vi "Main - On Load.vi"(8 "error in (no error)":errorcluster, 11 "Device Item Ref in":T1 format="%.0x") -> (0 "error out":errorcluster, 3 "Device Item Ref out":T1 format="%.0x")   [LabVIEW 2017, in "Scan Engine Custom Device.lvlib"]
uses:
  Scan Engine Custom Device.lvlib
  <vilib>/NI Veristand/Custom Device API/Custom Device Item Ref.ctl
  <vilib>/NI Veristand/Custom Device API/Custom Device Channel.ctl
  <vilib>/NI Veristand/Custom Device API/Custom Device Channel Type.ctl
  NationalInstruments.VeriStand.SystemDefinitionAPI
  Globals/Scan Engine GUIDs.vi
  Globals/Property Strings.vi
  <vilib>/NI Veristand/Custom Device Tools/Custom Device Utility Library/NI VeriStand - Search for All Items by GUID.vi
  <vilib>/NI Veristand/Custom Device API/Get Item Property (U32).vi
  Globals/String Constants.vi
  <vilib>/NI Veristand/Custom Device API/Set Item Property (Boolean).vi
  <vilib>/NI Veristand/Custom Device API/Custom Device API.lvlib
  <vilib>/NI Veristand/Custom Device Tools/Custom Device Utility Library/Custom Device Utility Library.lvlib
  Modules.lvlibp/RSI Module/RSI Module.lvclass
  Modules.lvlibp
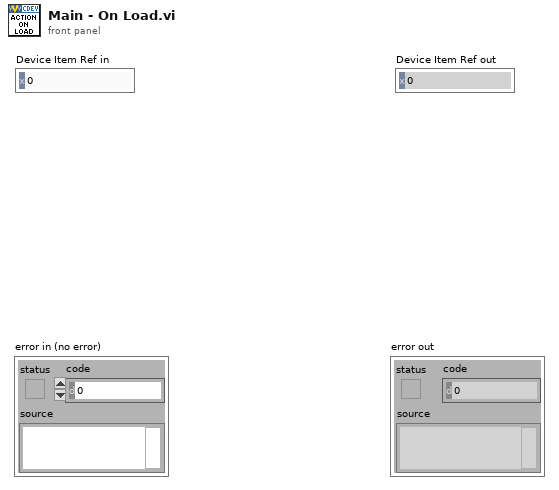
[diagram p1: front panel]
types:
  T1 = typedef "Custom Device API.lvlib/Custom Device Item Ref.ctl" = u64
  T2 = typedef "Custom Device API.lvlib/Custom Device Channel.ctl" = cluster{"Type":T3, "Units":string, "Default Value":dbl, "Faultable":bool, "Scalable":bool}
  T3 = typedef "Custom Device API.lvlib/Custom Device Channel Type.ctl" = enum16{"Input", "Output"}
  T4 = typedef "Modules.lvlibp/Custom Device API.lvlib/Custom Device Item Ref.ctl" = u64
  T5 = typedef "Modules.lvlibp/RSI Module.lvclass/Module Models.ctl" = enum16{"Empty", "NI 9201", "NI 9203", "NI 9205", "NI 9206", "NI 9207", "NI 9208", "NI 9211", "NI 9212", "NI 9213", "NI 9214", "NI 9215", "NI 9217", "NI 9219", "NI 9220", "NI 9221", "NI 9222", "NI 9223", "NI 9224", "NI 9225", "NI 9227", "NI 9229", "NI 9233", "NI 9234", "NI 9235", "NI 9236", "NI 9237", "NI 9239", "NI 9242", "NI 9244", "NI 9263", "NI 9264", "NI 9265", "NI 9266", "NI 9269", "NI 9375", "NI 9401", "NI 9402", "NI 9403", "NI 9411", "NI 9421", "NI 9422", "NI 9423", "NI 9425", "NI 9426", "NI 9435", "NI 9437", "NI 9472", "NI 9474", "NI 9475", "NI 9476", "NI 9477", "NI 9478", "NI 9481", "NI 9482", "NI 9485"}
  T6 = typedef "Modules.lvlibp/RSI Module.lvclass/Slot Settings.ctl" = cluster{"Slot":u32, "EtherCAT?":bool}
  T7 = typedef "Custom Device API.lvlib/Custom Device Item Info.ctl" = cluster{"Name":string, "Is Channel":bool, "GUID":string, "Is Waveform":bool}
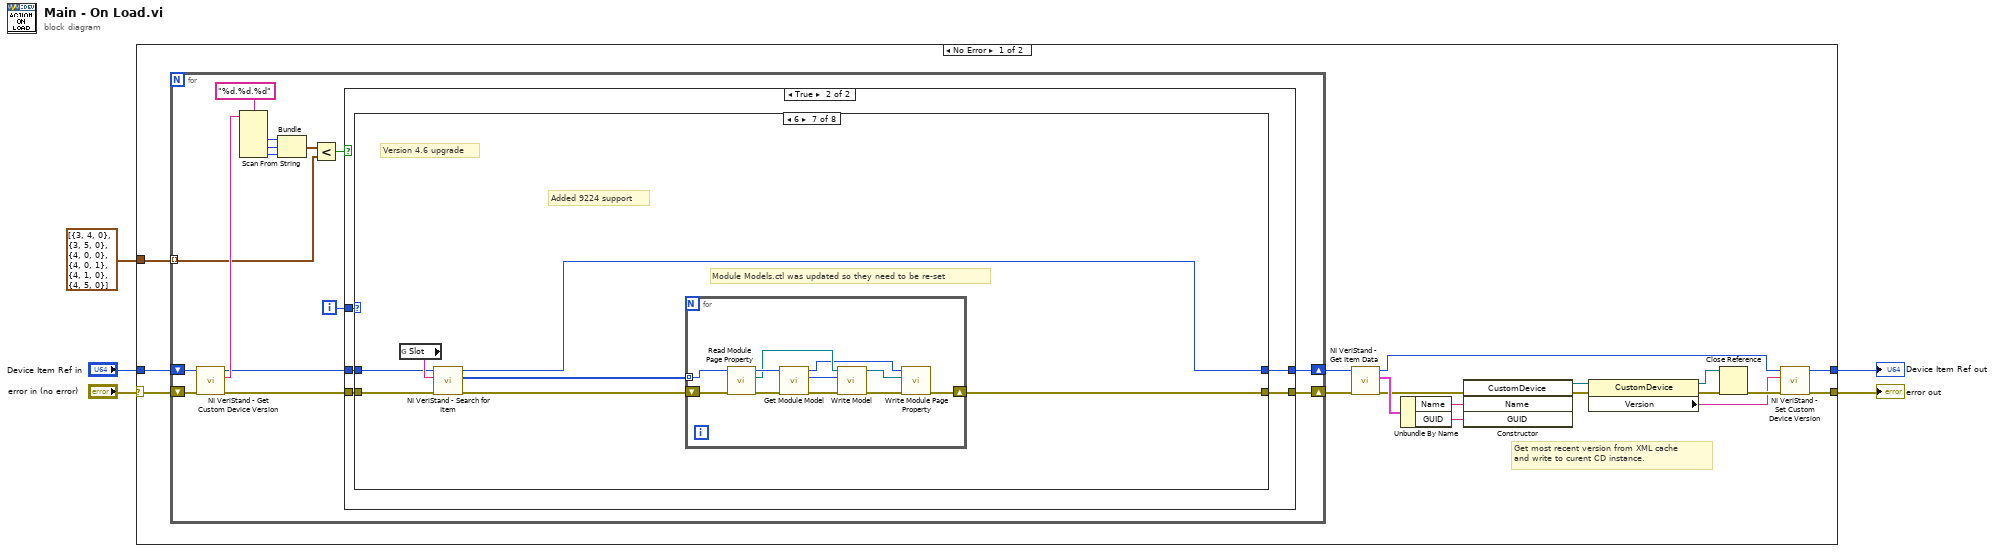
[diagram p0: block diagram]
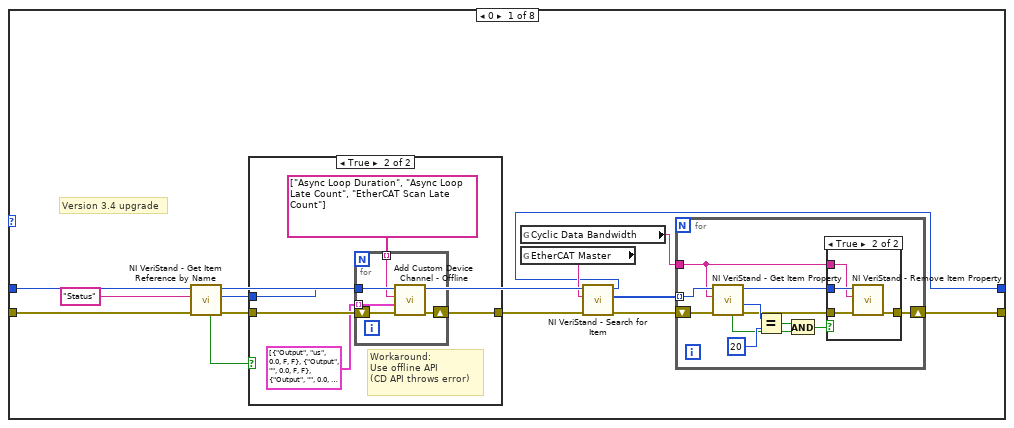
[diagram p3: hidden frame]
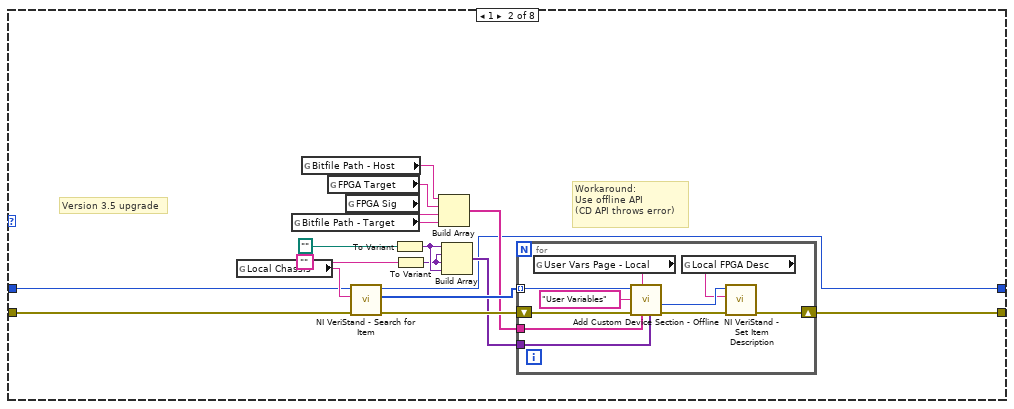
[diagram p6: hidden frame]
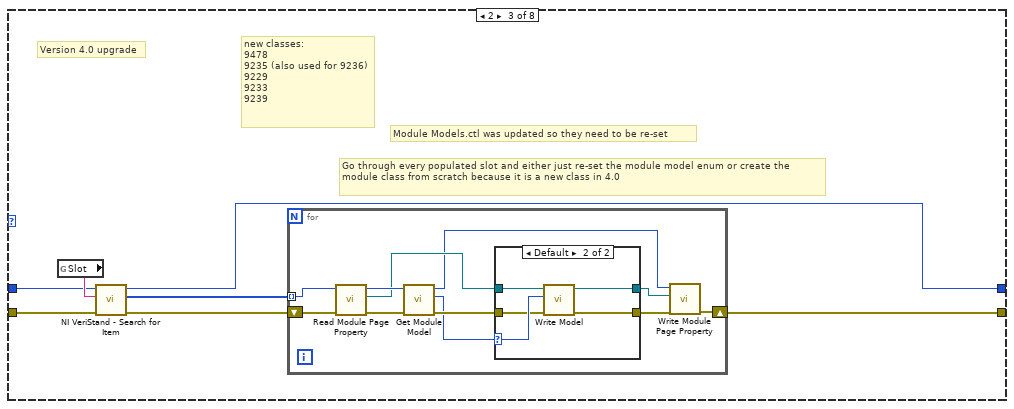
[diagram p7: hidden frame]
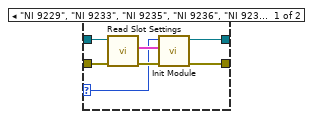
[diagram p8: hidden frame]
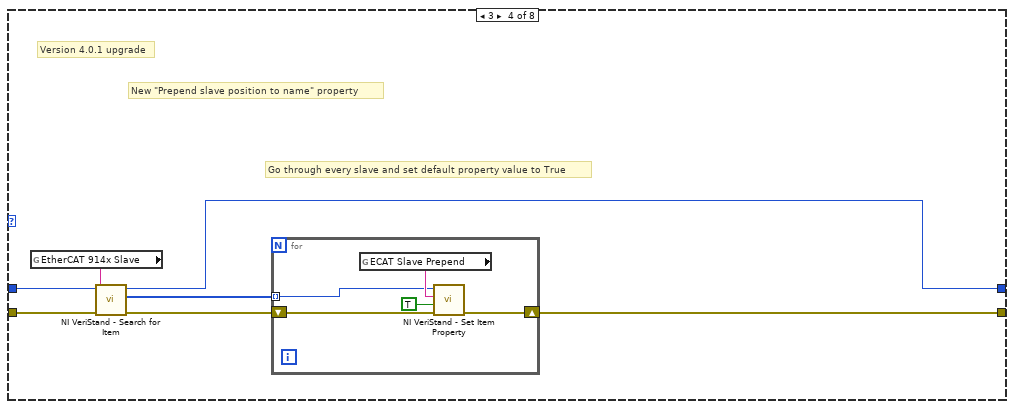
[diagram p9: hidden frame]
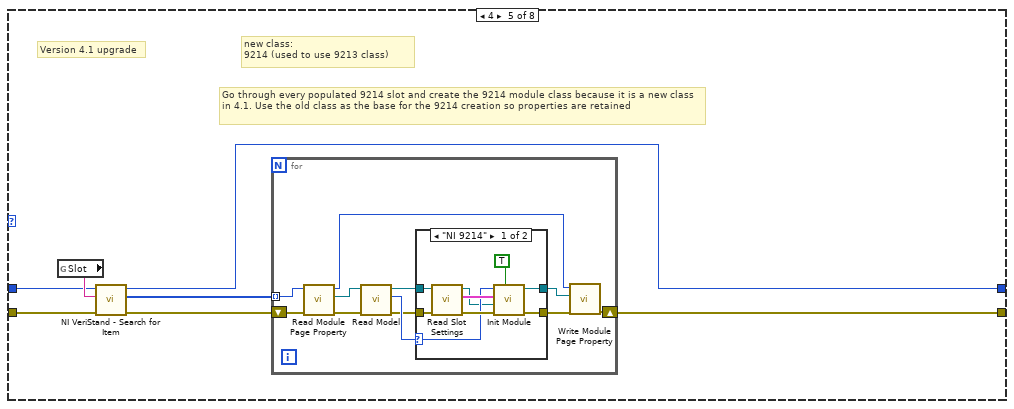
[diagram p10: hidden frame]
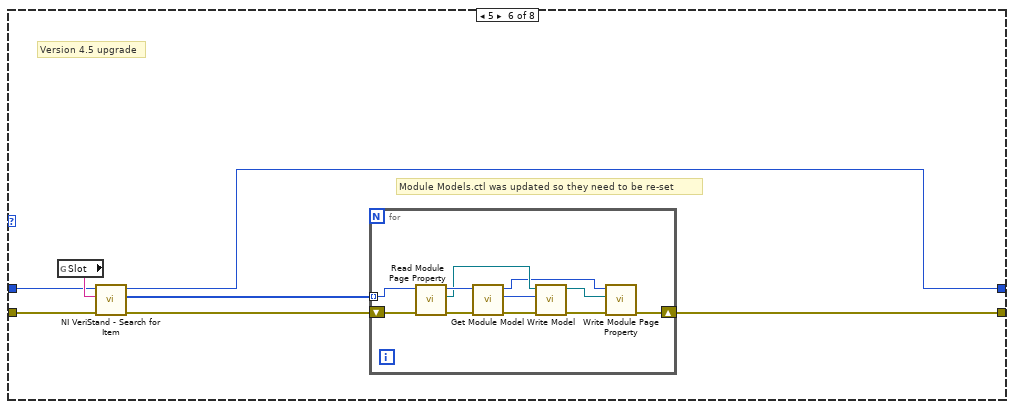
[diagram p12: hidden frame]
diagram:
  n1 = case shown="No Error" "error in (no error)" {
    selector: "error in (no error)" -> [w23 w224]
    tunnel: [w6 w224] -> w3
    tunnel: "Device Item Ref in" -> [w22 w223]
    tunnel: [w7 w223] -> w2
    tunnel: cluster{i32, i32, i32}[] [{3, 4, 0}, {3, 5, 0}, {4, 0, 0}, {4, 0, 1}, {4, 1, 0}, {4, 5, 0}] -> [w21 _]
    frame No Error {
      # "Get most recent version from XML cache\nand write to curent CD instance."
      n2 = for {
        shift-right: [w29] -> w19
        shift-left: w23 -> [w34]
        shift-right: [w27] -> w20
        shift-left: w22 -> [w33]
        tunnel: w21 -> [w24] mode=indexing
        i -> [w26]
        n3 = call <vilib>:"NI VeriStand - Get Custom Device Version.vi"("error in (no error)"=w34, "Device Ref in"=w33) -> ("error out"=w30:errorcluster, "Value"=w32:string, "Device Ref out"=w28:T1)  [unwired: 7 in]
        n4 = Scan From String(format string="%d.%d.%d", input string=w32) -> (output 1=w36:i32, output 2=w37:i32, output 3=w25:i32)  [unwired: 5 in, 3 out]
        n5 = Bundle(w36, w37, w25) -> (w38:cluster{i32, i32, i32})  [unwired: 1 in]
        n6 = Less?(x=w38, y=w24) -> (x < y?=w31:bool)
        n7 = case shown="True" w31 {
          tunnel: w30 -> [w40 w45]
          tunnel: [w40 w44] -> w29
          tunnel: w28 -> [w39 w41]
          tunnel: [w39 w42] -> w27
          tunnel: w26 -> [_ w43]
          frame False {
          }
          frame True {
            n8 = case shown="6" w43 {
              tunnel: w45 -> [w46 w89 w116 w146 w158 w187 w205 w222]
              tunnel: [w52 w88 w115 w145 w157 w186 w204 w222] -> w44
              tunnel: [w54 w87 w114 w144 w156 w185 w203 w221] -> w42
              tunnel: w41 -> [w47 w90 w117 w147 w159 w188 w206 w221]
              frame 0 {
                # "Version 3.4 upgrade"
                n9 = call <vilib>:"NI VeriStand - Get Item Reference by Name.vi"("error in (no error)"=w46, "Item Name"="Status" ("Section Name"), "Parent Ref in"=w47) -> ("error out"=w50:errorcluster, "Item Ref"=w49:T1, "Parent Ref out"=w58:T1, "Found"=w48:bool)  [unwired: 5 in]
                n10 = case shown="True" w48 {
                  tunnel: w49 -> [_ w65]
                  tunnel: w50 -> [w60 w64]
                  tunnel: [w60 w63] -> w59
                  frame False {
                  }
                  frame True {
                    # "Workaround:\nUse offline API\n(CD API throws error)"
                    n11 = for {
                      tunnel: w65 -> [w68]
                      shift-right: [w70] -> w63
                      shift-left: w64 -> [w69]
                      tunnel: T2[] [{"Type"=enum."Output", "Units"="us", "Default Value"=0.0, "Faultable"=FALSE, "Scalable"=FALSE}, {"Type"=enum."Output", "Units"="", "Default Value"=0.0, "Faultable"=FALSE, "Scalable"=FALSE}, {"Type"=enum."Output", "Units"="", "Default Value"=0.0, "Faultable"=FALSE, "Scalable"=FALSE}] -> [w66] mode=indexing
                      tunnel: string[] ["Async Loop Duration", "Async Loop Late Count", "EtherCAT Scan Late Count"] -> [w67] mode=indexing
                      n12 = call "Add Custom Device Channel - Offline.vi"("error in (no error)"=w69, "Channel"=w66, "Channel Name"=w67, "Parent Ref in"=w68) -> ("error out"=w70:errorcluster)  [unwired: 4 in, 3 out]
                    }
                  }
                }
                n13 = global read "Property Strings.vi" "Cyclic Data Bandwidth"() -> (w53:string)
                n14 = global read "Scan Engine GUIDs.vi" "EtherCAT Master"() -> (w57:string)
                n15 = call-poly <vilib>:"NI VeriStand - Search for Item.vi"("error in"=w59, "Item GUID"=w57, "Section Ref in"=w58) -> ("error out"=w55:errorcluster, "Item Refs"=w56:T1[], "Section Ref out"=w54:T1)  [unwired: 5 in, 1 out]
                n16 = for {
                  tunnel: w56 -> [w80] mode=indexing
                  shift-right: [w71] -> w52
                  shift-left: w55 -> [w81]
                  tunnel: w53 -> [w72]
                  n17 = call-poly <vilib>:"NI VeriStand - Get Item Property.vi"("error in (no error)"=w81, "Property Name"=w72, "Item Ref in"=w80) -> ("error out"=w74:errorcluster, "Value"=w79:u32, "Item Ref out"=w73:T1, "Found?"=w76:bool)  [unwired: 5 in]
                  n18 = Equal?(x=w79, y=u32 20 ("x")) -> (x = y?=w77:bool)
                  n19 = And(x=w77, y=w76) -> (x .and. y?=w75:bool)
                  n20 = case shown="True" w75 {
                    tunnel: w74 -> [w82 w85]
                    tunnel: w73 -> [_ w86]
                    tunnel: w72 -> [_ w84]
                    tunnel: [w82 w83] -> w71
                    frame False {
                    }
                    frame True {
                      n21 = call <vilib>:"NI VeriStand - Remove Item Property.vi"("error in (no error)"=w85, "Property Name"=w84, "Item Ref in"=w86) -> ("error out"=w83:errorcluster)  [unwired: 6 in, 2 out]
                    }
                  }
                }
              }
              frame 1 {
                # "Workaround:\nUse offline API\n(CD API throws error)"
                # "Version 3.5 upgrade"
                n22 = global read "Scan Engine GUIDs.vi" "Local Chassis"() -> (w101:string)
                n23 = global read "Property Strings.vi" "Bitfile Path - Target"() -> (w94:string)
                n24 = global read "Property Strings.vi" "Bitfile Path - Host"() -> (w97:string)
                n25 = global read "Property Strings.vi" "FPGA Target"() -> (w96:string)
                n26 = global read "Property Strings.vi" "FPGA Sig"() -> (w95:string)
                n27 = call-poly <vilib>:"NI VeriStand - Search for Item.vi"("error in"=w89, "Item GUID"=w101, "Section Ref in"=w90) -> ("error out"=w103:errorcluster, "Item Refs"=w102:T1[], "Section Ref out"=w87:T1)  [unwired: 5 in, 1 out]
                n28 = To Variant(anything=path "") -> (Variant=w93:variant)
                n29 = To Variant(anything="") -> (Variant=w91:variant)
                n30 = Build Array(w97, w96, w95, w94) -> (w99:string[])
                n31 = Build Array(w93, w91, w91, w93) -> (w100:variant[])
                n32 = for {
                  tunnel: w99 -> [w112]
                  tunnel: w100 -> [w111]
                  shift-right: [w106] -> w88
                  shift-left: w103 -> [w113]
                  tunnel: w102 -> [w110] mode=indexing
                  n33 = global read "Scan Engine GUIDs.vi" "User Vars Page - Local"() -> (w109:string)
                  n34 = call "Add Custom Device Section - Offline.vi"("Property Values"=w111, "Property names"=w112, "GUID (Default Section)"=w109, "error in (no error)"=w113, "Section Name"="User Variables", "Parent Ref in"=w110) -> ("error out"=w107:errorcluster, "Section Ptr"=w105:T1)  [unwired: 2 in, 2 out]
                  n35 = global read "String Constants.vi" "Local FPGA Desc"() -> (w104:string)
                  n36 = call <vilib>:"NI VeriStand - Set Item Description.vi"("error in (no error)"=w107, "Description"=w104, "Item Ref in"=w105) -> ("error out"=w106:errorcluster)  [unwired: 6 in, 2 out]
                }
              }
              frame 2 {
                # "new classes:\n9478\n9235 (also used for 9236)\n9229\n9233\n9239"
                # "Go through every populated slot and either just re-set the module model enum or create the module class from scratch because it is a new class in 4.0"
                # "Module Models.ctl was updated so they need to be re-set"
                # "Version 4.0 upgrade"
                n37 = global read "Scan Engine GUIDs.vi" "Slot"() -> (w118:string)
                n38 = call-poly <vilib>:"NI VeriStand - Search for Item.vi"("error in"=w116, "Item GUID"=w118, "Section Ref in"=w117) -> ("error out"=w120:errorcluster, "Item Refs"=w119:T1[], "Section Ref out"=w114:T1)  [unwired: 5 in, 1 out]
                n39 = for {
                  shift-right: [w131] -> w115
                  shift-left: w120 -> [w127]
                  tunnel: w119 -> [w128] mode=indexing
                  n40 = call "Read Module Page Property.vi"("error in (no error)"=w127, "Node Ptr In"=w128) -> ("error out"=w130:errorcluster, "RSI Module"=w125:refnum<class "RSI Module.lvclass">, "Node Ptr Out"=w129:T4)  [unwired: 7 in]
                  n41 = call "Get Module Model.vi"("error in (no error)"=w130, "Item Ref in"=w129) -> ("error out"=w122:errorcluster, "Module"=w121:T5, "Item Ref out"=w123:T1)  [unwired: 7 in]
                  n42 = case shown="Default" w121 {
                    selector: w121 -> [w135 w142]
                    tunnel: [w134 w143] -> w126
                    tunnel: w125 -> [w136 w141]
                    tunnel: [w133 w140] -> w124
                    tunnel: w122 -> [w132 w139]
                    frame "NI 9229", "NI 9233", "NI 9235", "NI 9236", "NI 9239", "NI 9478" {
                      n43 = call "Read Slot Settings.vi"("error in (no error)"=w132, "RSI Module in"=w136) -> ("error out"=w137:errorcluster, "Slot Settings"=w138:T6)  [unwired: 7 in, 1 out]
                      n44 = call "Init Module.vi"("error in (no error)"=w137, "Slot Settings"=w138, "Module Model"=w135) -> ("error out"=w134:errorcluster, "RSI Module out"=w133:refnum<class "RSI Module.lvclass">)  [unwired: 7 in]
                    }
                    frame Default {
                      n45 = call "Write Model.vi"("error in (no error)"=w139, "Model"=w142, "RSI Module in"=w141) -> ("error out"=w143:errorcluster, "RSI Module out"=w140:refnum<class "RSI Module.lvclass">)  [unwired: 7 in]
                    }
                  }
                  n46 = call "Write Module Page Property.vi"("error in (no error)"=w126, "RSI Module"=w124, "Node Ptr In"=w123) -> ("error out"=w131:errorcluster)  [unwired: 6 in, 2 out]
                }
              }
              frame 3 {
                # "New \"Prepend slave position to name\" property"
                # "Go through every slave and set default property value to True"
                # "Version 4.0.1 upgrade"
                n47 = global read "Scan Engine GUIDs.vi" "EtherCAT 914x Slave"() -> (w148:string)
                n48 = call-poly <vilib>:"NI VeriStand - Search for Item.vi"("error in"=w146, "Item GUID"=w148, "Section Ref in"=w147) -> ("error out"=w150:errorcluster, "Item Refs"=w149:T1[], "Section Ref out"=w144:T1)  [unwired: 5 in, 1 out]
                n49 = for {
                  shift-right: [w151] -> w145
                  shift-left: w150 -> [w155]
                  tunnel: w149 -> [w153] mode=indexing
                  n50 = global read "Property Strings.vi" "ECAT Slave Prepend"() -> (w154:string)
                  n51 = call-poly <vilib>:"NI VeriStand - Set Item Property.vi"("error in (no error)"=w155, "Value"=TRUE, "Property Name"=w154, "Item Ref in"=w153) -> ("error out"=w151:errorcluster)  [unwired: 5 in, 2 out]
                }
              }
              frame 4 {
                # "new class:\n9214 (used to use 9213 class)"
                # "Go through every populated 9214 slot and create the 9214 module class because it is a new class in 4.1. Use the old class as the base for the 9214 creation so properties are retained"
                # "Version 4.1 upgrade"
                n52 = global read "Scan Engine GUIDs.vi" "Slot"() -> (w160:string)
                n53 = call-poly <vilib>:"NI VeriStand - Search for Item.vi"("error in"=w158, "Item GUID"=w160, "Section Ref in"=w159) -> ("error out"=w162:errorcluster, "Item Refs"=w161:T1[], "Section Ref out"=w156:T1)  [unwired: 5 in, 1 out]
                n54 = for {
                  shift-right: [w173] -> w157
                  shift-left: w162 -> [w171]
                  tunnel: w161 -> [w172] mode=indexing
                  n55 = call "Read Module Page Property.vi"("error in (no error)"=w171, "Node Ptr In"=w172) -> ("error out"=w168:errorcluster, "RSI Module"=w167:refnum<class "RSI Module.lvclass">, "Node Ptr Out"=w163:T4)  [unwired: 7 in]
                  n56 = call "Read Model.vi"("error in (no error)"=w168, "RSI Module in"=w167) -> ("error out"=w164:errorcluster, "Model"=w165:T5, "RSI Module out"=w166:refnum<class "RSI Module.lvclass">)  [unwired: 7 in]
                  n57 = case shown="\"NI 9214\"" w165 {
                    selector: w165 -> [w180 _]
                    tunnel: w164 -> [w179 w184]
                    tunnel: [w175 w184] -> w170
                    tunnel: w166 -> [w176 w183]
                    tunnel: [w174 w183] -> w169
                    frame "NI 9214" {
                      n58 = call "Read Slot Settings.vi"("error in (no error)"=w179, "RSI Module in"=w176) -> ("error out"=w181:errorcluster, "Slot Settings"=w182:T6, "RSI Module out"=w177:refnum<class "RSI Module.lvclass">)  [unwired: 7 in]
                      n59 = call "Init Module.vi"("Create from class input? (F)"=TRUE, "error in (no error)"=w181, "RSI Module in"=w177, "Slot Settings"=w182, "Module Model"=w180) -> ("error out"=w175:errorcluster, "RSI Module out"=w174:refnum<class "RSI Module.lvclass">)  [unwired: 5 in]
                    }
                    frame Default {
                    }
                  }
                  n60 = call "Write Module Page Property.vi"("error in (no error)"=w170, "RSI Module"=w169, "Node Ptr In"=w163) -> ("error out"=w173:errorcluster)  [unwired: 6 in, 2 out]
                }
              }
              frame 5 {
                # "Module Models.ctl was updated so they need to be re-set"
                # "Version 4.5 upgrade"
                n61 = global read "Scan Engine GUIDs.vi" "Slot"() -> (w189:string)
                n62 = call-poly <vilib>:"NI VeriStand - Search for Item.vi"("error in"=w187, "Item GUID"=w189, "Section Ref in"=w188) -> ("error out"=w191:errorcluster, "Item Refs"=w190:T1[], "Section Ref out"=w185:T1)  [unwired: 5 in, 1 out]
                n63 = for {
                  shift-right: [w202] -> w186
                  shift-left: w191 -> [w198]
                  tunnel: w190 -> [w199] mode=indexing
                  n64 = call "Read Module Page Property.vi"("error in (no error)"=w198, "Node Ptr In"=w199) -> ("error out"=w201:errorcluster, "RSI Module"=w194:refnum<class "RSI Module.lvclass">, "Node Ptr Out"=w200:T4)  [unwired: 7 in]
                  n65 = call "Get Module Model.vi"("error in (no error)"=w201, "Item Ref in"=w200) -> ("error out"=w197:errorcluster, "Module"=w196:T5, "Item Ref out"=w192:T1)  [unwired: 7 in]
                  n66 = call "Write Model.vi"("error in (no error)"=w197, "Model"=w196, "RSI Module in"=w194) -> ("error out"=w195:errorcluster, "RSI Module out"=w193:refnum<class "RSI Module.lvclass">)  [unwired: 7 in]
                  n67 = call "Write Module Page Property.vi"("error in (no error)"=w195, "RSI Module"=w193, "Node Ptr In"=w192) -> ("error out"=w202:errorcluster)  [unwired: 6 in, 2 out]
                }
              }
              frame 6 {
                # "Added 9224 support"
                # "Module Models.ctl was updated so they need to be re-set"
                # "Version 4.6 upgrade"
                n68 = global read "Scan Engine GUIDs.vi" "Slot"() -> (w207:string)
                n69 = call-poly <vilib>:"NI VeriStand - Search for Item.vi"("error in"=w205, "Item GUID"=w207, "Section Ref in"=w206) -> ("error out"=w209:errorcluster, "Item Refs"=w208:T1[], "Section Ref out"=w203:T1)  [unwired: 5 in, 1 out]
                n70 = for {
                  shift-right: [w220] -> w204
                  shift-left: w209 -> [w216]
                  tunnel: w208 -> [w217] mode=indexing
                  n71 = call "Read Module Page Property.vi"("error in (no error)"=w216, "Node Ptr In"=w217) -> ("error out"=w219:errorcluster, "RSI Module"=w212:refnum<class "RSI Module.lvclass">, "Node Ptr Out"=w218:T4)  [unwired: 7 in]
                  n72 = call "Get Module Model.vi"("error in (no error)"=w219, "Item Ref in"=w218) -> ("error out"=w215:errorcluster, "Module"=w214:T5, "Item Ref out"=w210:T1)  [unwired: 7 in]
                  n73 = call "Write Model.vi"("error in (no error)"=w215, "Model"=w214, "RSI Module in"=w212) -> ("error out"=w213:errorcluster, "RSI Module out"=w211:refnum<class "RSI Module.lvclass">)  [unwired: 7 in]
                  n74 = call "Write Module Page Property.vi"("error in (no error)"=w213, "RSI Module"=w211, "Node Ptr In"=w210) -> ("error out"=w220:errorcluster)  [unwired: 6 in, 2 out]
                }
              }
              frame Default {
              }
            }
          }
        }
      }
      n75 = call <vilib>:"NI VeriStand - Get Item Data.vi"("error in (no error)"=w19, "Item Ref in"=w20) -> ("error out"=w15:errorcluster, "Item Info"=w18:T7, "Item Ref out"=w8:T1)  [unwired: 6 in, 1 out]
      n76 = Unbundle By Name(w18) -> ("Name"=w17:string, "GUID"=w16:string)
      n77 = constructor class="CustomDevice"(error in=w15, "Name"=w17, "GUID"=w16) -> (reference out=w14:refnum<k24>, error out=w13:errorcluster)  [unwired: 2 in, 3 out]
      n78 = property class="CustomDevice"(reference=w14, error in=w13) -> (reference out=w11:refnum<k24>, error out=w12:errorcluster, "Version"=w9:string)
      n79 = Close Reference(reference=w11, error in (no error)=w12) -> (error out=w10:errorcluster)
      n80 = call <vilib>:"NI VeriStand - Set Custom Device Version.vi"("error in (no error)"=w10, "Value"=w9, "Device Ref in"=w8) -> ("error out"=w6:errorcluster, "Device Ref out"=w7:T1)  [unwired: 7 in]
    }
    frame Error {
    }
  }
  "error out" <- w3
  "Device Item Ref out" <- w2
